vi "Write.vi"(10 "Time Stamp":timestamp, 11 "Time Stamp in":refnum<class "Time Stamp.lvclass">) -> (3 "Time Stamp out":refnum<class "Time Stamp.lvclass">)   [LabVIEW 2020, in "Data.lvlib" / "Time Stamp.lvclass"]
doc: "Write Time Stamp."
uses:
  Time Stamp.lvclass
  Time Stamp.lvclass/Time Stamp.ctl
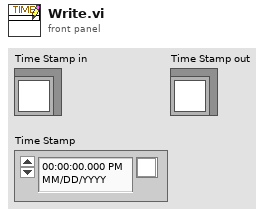
[diagram p1: front panel]
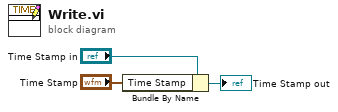
[diagram p0: block diagram]
diagram:
  n1 = Bundle By Name(cluster="Time Stamp in", "Time Stamp"="Time Stamp") -> (→"Time Stamp out":refnum<class "Time Stamp.lvclass">)
